vi "Write Parabolic Params.vi"(9 "low":dbl, 10 "high":dbl, 11 "Parabolic Setpoint in":refnum<class "Parabolic Setpoint.lvclass">) -> (3 "Parabolic Setpoint out":refnum<class "Parabolic Setpoint.lvclass">)   [LabVIEW 2020, in "Parabolic Setpoint.lvclass"]
uses:
  Parabolic Setpoint.lvclass
  Parabolic Setpoint.lvclass/Parabolic Setpoint.ctl
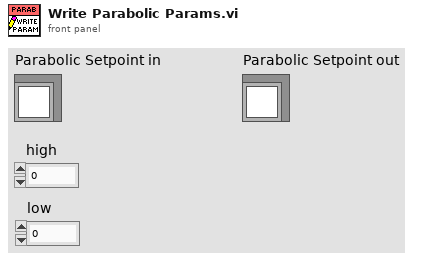
[diagram p1: front panel]
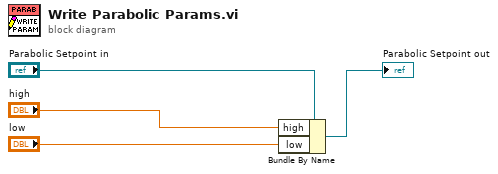
[diagram p0: block diagram]
diagram:
  n1 = Bundle By Name(cluster="Parabolic Setpoint in", "high"="high", "low"="low") -> (→"Parabolic Setpoint out":refnum<class "Parabolic Setpoint.lvclass">)
